vi "CSP_addTrainingData.vi"(8 "error in":errorcluster, 10 "NumberOfClasses":i32, 11 "CSP.lvclass in":refnum<class "CSP.lvclass">) -> (0 "error out":errorcluster, 3 "CSP.lvclass out":refnum<class "CSP.lvclass">)   [LabVIEW 2016, in "Spatial Pattern Filter.lvlib" / "CSP.lvclass"]
uses:
  CSP.lvclass
  CSP.lvclass/CSP.ctl
panel:
  # "This VI is a part of BCI Design library, http://www.ru-bci.org \nCopyright © 2020, Sotnikov Peter, All rights reserved. License: CC BY-NC 4.0"
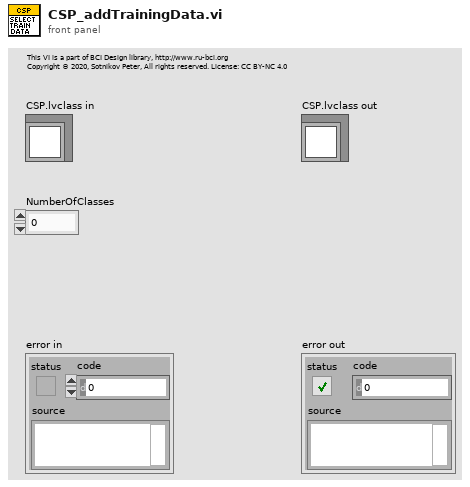
[diagram p1: front panel]
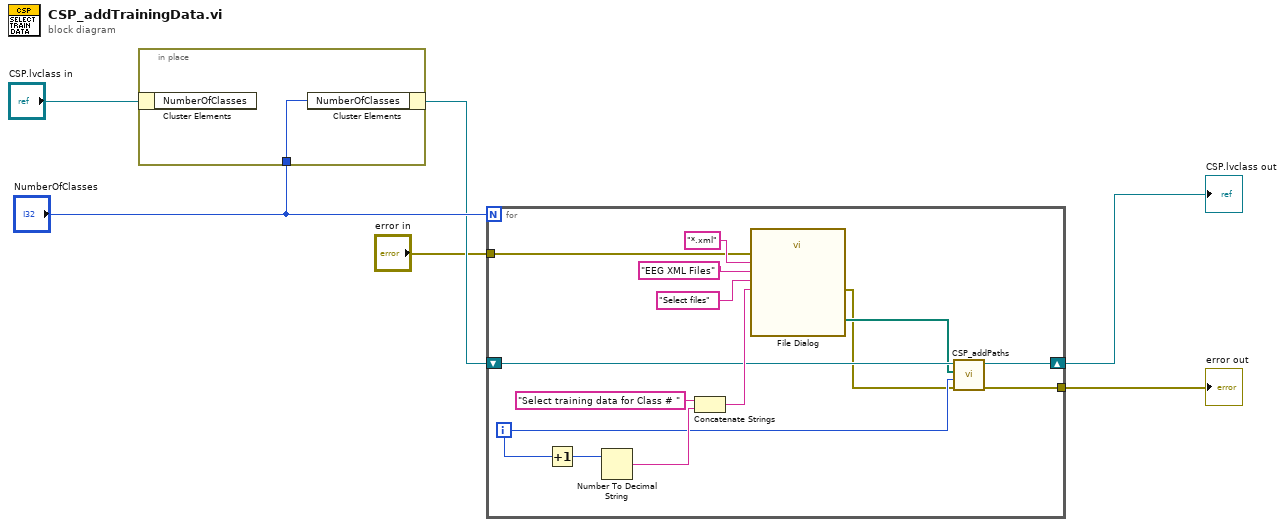
[diagram p0: block diagram]
diagram:
  n1 = in-place {
    in-place-border: "NumberOfClasses" -> [w7]
    n2 = in-place-cluster #1("CSP.lvclass in") -> ()  [unwired: 1 out]
    n3 = in-place-cluster #1("NumberOfClasses"=w7) -> (w4:refnum<class "CSP.lvclass">)
  }
  n4 = for {
    N: "NumberOfClasses" -> [_]
    shift-right: [w10] -> w2
    shift-left: w4 -> [w13]
    tunnel: "error in" -> [w14]
    tunnel: [w8] -> w1
    i -> [w11]
    n5 = Increment(x=w11) -> (x+1=w18:i32)
    n6 = Number To Decimal String(number=w18) -> (decimal integer string=w15:string)  [unwired: 1 in]
    n7 = Concatenate Strings("Select training data for Class # " ("string"), w15) -> (w17:string)
    n8 = call "File Dialog"("prompt"=w17, "button label"="Select files", "error in"=w14, "pattern (all files)"="*.xml", "pattern label"="EEG XML Files") -> ("selected paths"=w12:path[], "error out"=w9:errorcluster)  [unwired: 7 in, 2 out]
    n9 = call "CSP_addPaths.vi"("error in"=w9, "ClassId"=w11, "Selected Paths"=w12, "CSP.lvclass in"=w13) -> ("error out"=w8:errorcluster, "CSP.lvclass out"=w10:refnum<class "CSP.lvclass">)  [unwired: 6 in]
  }
  "CSP.lvclass out" <- w2
  "error out" <- w1
